vi "(SubVI)_Control_Save_Controller_bin_MultiSite.vi"(10 "Input cluster":T1, 11 "refnum in":refnum<file>) -> (0 "error out":errorcluster, 3 "refnum out":refnum<file>)   [LabVIEW 2019]
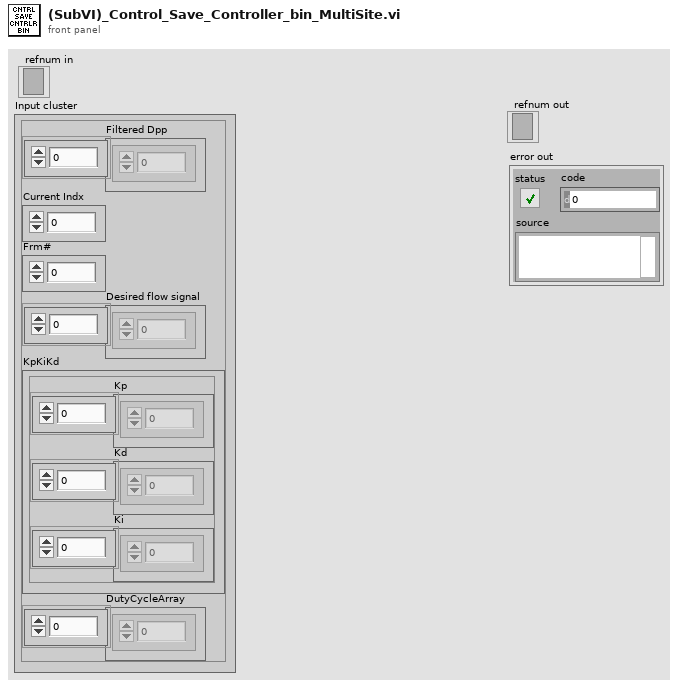
[diagram p1: front panel]
types:
  T1 = cluster{"Filtered Dpp":dbl[], "Current Indx":dbl, "Frm#":dbl, "Desired flow signal":dbl[], "KpKiKd":cluster{"Kp":dbl[], "Kd":dbl[], "Ki":dbl[]}, "DutyCycleArray":dbl[]}
  T2 = enum16{"big-endian, network order", "native, host order", "little-endian"}
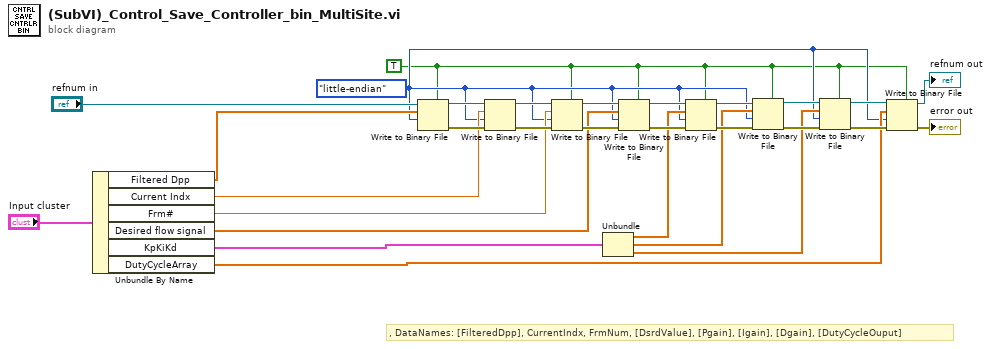
[diagram p0: block diagram]
diagram:
  w2 = T2."little-endian" ("byte order (0:big-endian, network order)")
  w1 = TRUE ("prepend array or string size? (T)")
  # ", DataNames: [FilteredDpp], CurrentIndx, FrmNum, [DsrdValue], [Pgain], [Igain], [Dgain], [DutyCycleOuput]"
  n1 = Unbundle By Name("Input cluster") -> ("Filtered Dpp"=w18:dbl[], "Current Indx"=w13:dbl, "Frm#"=w12:dbl, "Desired flow signal"=w11:dbl[], "KpKiKd"=w9:cluster{"Kp":dbl[], "Kd":dbl[], "Ki":dbl[]}, "DutyCycleArray"=w10:dbl[])
  n2 = Write to Binary File(file (use dialog)="refnum in", data=w18, 5:w1, 9:w2) -> (refnum out=w16:refnum<file>, error out=w17:errorcluster)  [unwired: 2 in, 1 out]
  n3 = Write to Binary File(file (use dialog)=w16, data=w13, error in=w17, 9:w2) -> (refnum out=w14:refnum<file>, error out=w15:errorcluster)  [unwired: 2 in, 1 out]
  n4 = Write to Binary File(file (use dialog)=w14, data=w12, error in=w15, 5:w1, 9:w2) -> (refnum out=w26:refnum<file>, error out=w23:errorcluster)  [unwired: 1 in, 1 out]
  n5 = Unbundle(w9) -> ("Kp"=w8:dbl[], "Kd"=w7:dbl[], "Ki"=w6:dbl[])
  n6 = Write to Binary File(file (use dialog)=w26, data=w11, error in=w23, 5:w1, 9:w2) -> (refnum out=w25:refnum<file>, error out=w22:errorcluster)  [unwired: 1 in, 1 out]
  n7 = Write to Binary File(file (use dialog)=w25, data=w8, error in=w22, 5:w1, 9:w2) -> (refnum out=w5:refnum<file>, error out=w21:errorcluster)  [unwired: 1 in, 1 out]
  n8 = Write to Binary File(file (use dialog)=w5, data=w7, 5:w1, 9:w2) -> (refnum out=w4:refnum<file>)  [unwired: 2 in, 2 out]
  n9 = Write to Binary File(file (use dialog)=w4, data=w6, 5:w1, 9:w2) -> (refnum out=w3:refnum<file>)  [unwired: 2 in, 2 out]
  n10 = Write to Binary File(file (use dialog)=w3, data=w10, error in=w21, 5:w1, 9:w2) -> (refnum out=→"refnum out":refnum<file>, error out=→"error out":errorcluster)  [unwired: 1 in, 1 out]
